vi "Initiate and Generate Time (Multi).vi"(0 "niUsrpRio Sessions":T3[](array[typedef]) {"Daughterboard Clock Rate" format="%#.3pHz"; "FPGA Data Clock Rate" format="%#.3pHz"; "Data Clock Rate" format="%#.3pHz"; "Characterization Data"."Frequencies [Hz]" format="%#_6p"; "EEPROM Characterization Header"."Pointer to Device Data Header" format="%x"; "EEPROM Characterization Header"."Checksum" format="%x"; "Device Data Header"."Pointer to Characterization Data" format="%x"; "Device Data Header"."Checksum" format="%x"; "EEPROM Header"."Pointer to User Header" format="%x"; "EEPROM Header"."Pointer to Factory Header" format="%x"; "EEPROM Header"."Product Code" format="%x"; "EEPROM Header"."Checksum" format="%x"}, 1 "tx channels":T1[](array[typedef]) {"tx.coerced configurations"."coerced sample rates" format="%#.3pS/s"; "tx.coerced configurations"."coerced levels" format="%#.3gdBm"; "tx.coerced configurations"."coerced lo frequencies" format="%#.3pHz"; "tx.coerced configurations"."coerced frequencies" format="%#.3pHz"; "tx config"."channel configuration"."channel configuration"."frequency" format="%#.3pHz"; "tx config"."channel configuration"."channel configuration"."lo frequency" format="%#.3pHz"; "tx config"."channel configuration"."channel configuration"."level" format="%#_gdBm"; "tx config"."tone frequency" format="%#.3pHz"; "tx config"."sample rate" format="%#.3pS/s"}, 5 "first iteration":bool, 7 "start trigger time":timestamp, 11 "error in":errorcluster) -> (4 "niUsrpRio Sessions (out)":T3[](array[typedef]) {"Daughterboard Clock Rate" format="%#.3pHz"; "FPGA Data Clock Rate" format="%#.3pHz"; "Data Clock Rate" format="%#.3pHz"; "Characterization Data"."Frequencies [Hz]" format="%#_6p"; "EEPROM Characterization Header"."Pointer to Device Data Header" format="%x"; "EEPROM Characterization Header"."Checksum" format="%x"; "Device Data Header"."Pointer to Characterization Data" format="%x"; "Device Data Header"."Checksum" format="%x"; "EEPROM Header"."Pointer to User Header" format="%x"; "EEPROM Header"."Pointer to Factory Header" format="%x"; "EEPROM Header"."Product Code" format="%x"; "EEPROM Header"."Checksum" format="%x"}, 15 "error out":errorcluster)   [LabVIEW 2020]
doc: "Writes baseband waveform to the device then initiates generation.\n\nVIs that must execute before this VI:\nOpen and Configure.vi\n\n<B>Input Parameters</B>\n\n<B>niUsrpRio Session</B> is the object created by the Open VI and used as the session handle for the USRP RIO design library.\n\n<B>first iteration</B> is used to determine if the device needs to be triggered. If this VI is in a loop, wire the iteration count to Equals Zero and then to this terminal. If this VI is not in a loop, wire a TRUE constant to this this terminal.\n\n<B>start trigger time</B> specifies the absolute time to initiate the start trigger. Only applies when the start trigger is set to Future Event.\n\n<B>error in</B> describes error conditions that occur before this node runs. This input provides standard 'error in' functionality.\n\n<B>Output Parameters</B>\n\n<B>niUsrpRio Session (out)</B> is the niUsrpRio session used in all subsequent USRP RIO design library host VIs.\n\n<B>error out</B> contains error information. This output provides standard 'error out' functionality."
uses:
  <instrlib>/niUsrpRio/Config/v1/Host/Public/niUsrpRio Session.ctl
  <instrlib>/_niInstr/Register Bus/v0/Host/Public/Register Bus Session.ctl
  <instrlib>/_niInstr/Register Bus/v0/Host/Private/Session Data.ctl
  <instrlib>/niUsrpRio/Config/v1/Host/Private/DB Queue Reference.ctl
  <instrlib>/niUsrpRio/Config/v1/Host/Private/Daughterboard Data.ctl
  <instrlib>/niUsrpRio/Config/v1/Host/Private/ATR state data.ctl
  <instrlib>/niUsrpRio/Config/v1/Host/Private/Antenna Configuration.ctl
  <instrlib>/niUsrpRio/Config/v1/Host/Private/CPLD Power Mode.ctl
  <instrlib>/niUsrpRio/Config/v1/Host/Public/EEPROM Header.ctl
  <instrlib>/niUsrpRio/Config/v1/Host/Public/EEPROM Device Data Header.ctl
  <instrlib>/niUsrpRio/Config/v1/Host/Public/EEPROM Characterization Header.ctl
  <instrlib>/niUsrpRio/Config/v1/Host/Public/Characterization Data.ctl
  <instrlib>/niUsrpRio/Config/v1/Host/Public/IQ Imbalance.ctl
  Tx Channels.ctl
  Start Trigger.ctl
  Write Tx Data (I16 multi).vi
  <instrlib>/_niInstr/Register Bus/v0/Host/niInstr Register Bus v0 Host.lvlib
  <instrlib>/niUsrpRio/Config/v1/Host/niUsrpRio Config v1 Host.lvlib
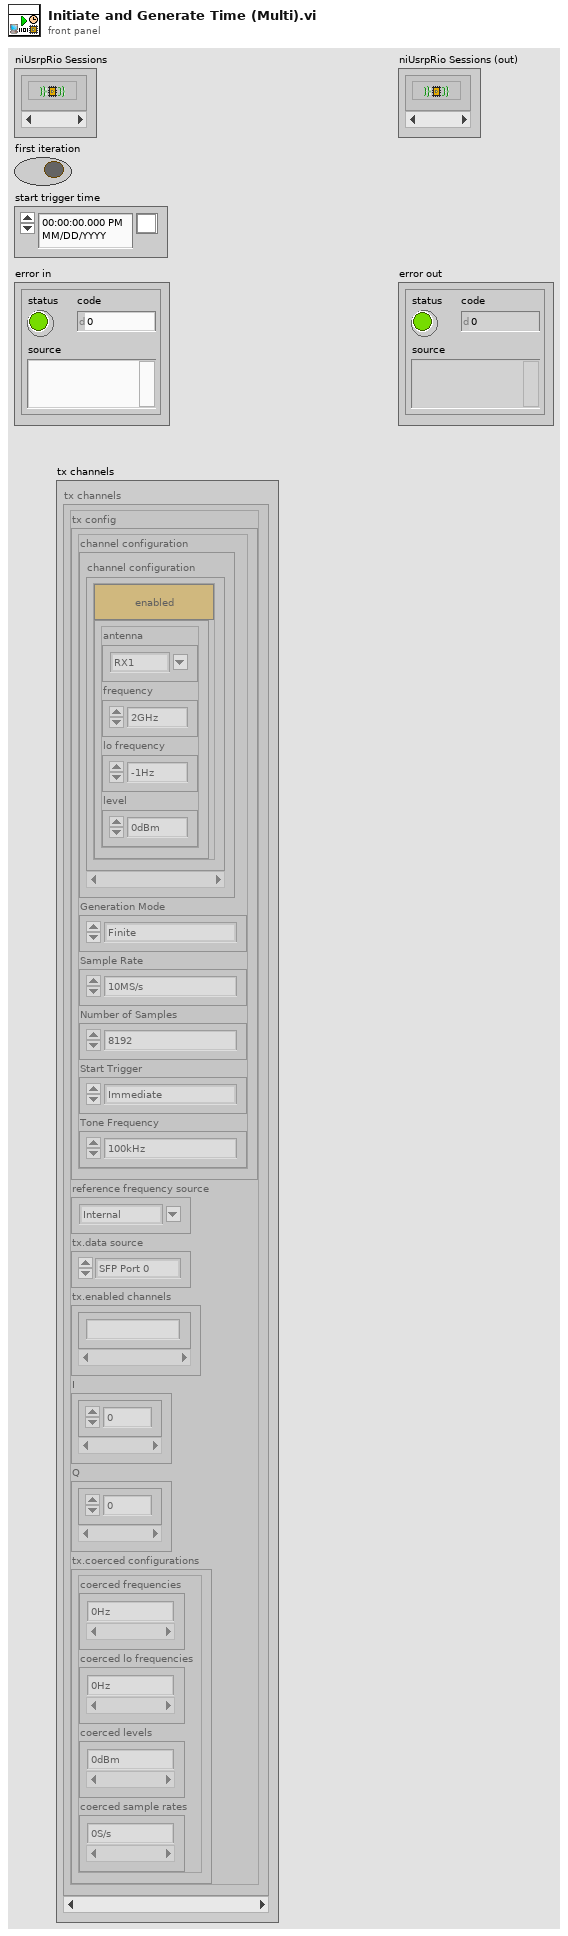
[diagram p1: front panel]
types:
  T1 = typedef "Tx Channels.ctl" = cluster{"tx config":cluster{"channel configuration":cluster{"channel enable":bool, "channel configuration":cluster{"antenna":string, "frequency":dbl, "lo frequency":dbl, "level":dbl}}[], "transfer mode":enum16{"Finite", "Continuous"}, "sample rate":dbl, "number of samples":u32, "start trigger":T2, "tone frequency":dbl}, "reference frequency source":string, "tx.data source":enum16{"SFP Port 0", "SFP Port 1", "Host"}, "tx.enabled channels":string[], "I":i16[], "Q":i16[], "tx.coerced configurations":cluster{"coerced frequencies":dbl[], "coerced lo frequencies":dbl[], "coerced levels":dbl[], "coerced sample rates":dbl[]}}
  T2 = typedef "Start Trigger.ctl" = enum8{"Software", "Digital Edge", "Rx Start Trigger", "Tx Start Trigger", "Immediate", "Future Time Event"}
  T3 = typedef "niUsrpRio Config v1 Host.lvlib/niUsrpRio Session.ctl" = cluster{"FPGA Interface":refnum<k20>, "RIO Interface Number":u32, "Data Clock Rate":u32, "FPGA Data Clock Rate":u32, "Global Settings Register Bus":T4, "Radio 0 Settings Register Bus":T4, "Radio 1 Settings Register Bus":T4, "Radio Settings Bus Semaphore":T5, "DB Queues":T6[], "Characterization Data Valid?":bool, "EEPROM Header":T7, "Device Data Header":T8, "EEPROM Characterization Header":T9, "Characterization Data":T10[], "FPGA Current Version":u32, "FPGA Oldest Compatible Version":u32, "Fixed Logic Current Version":u32, "Fixed Logic Oldest Compatible Version":u32, "FPGA Radio Settings Bus Current Version":u32, "FPGA Radio Settings Bus Oldest Compatible Version":u32, "FPGA Board Config Current Version":u32, "FPGA Board Config Oldest Compatible Version":u32, "Daughterboard Clock Rate":u32, "daughterboard configuration session handles":u64[]}
  T4 = typedef "niInstr Register Bus v0 Host.lvlib/Register Bus Session.ctl" = refnum<queue>
  T5 = typedef "Semaphore RefNum" = refnum<k1>
  T6 = typedef "niUsrpRio Config v1 Host.lvlib/DB Queue Reference.ctl" = refnum<queue>
  T7 = typedef "niUsrpRio Config v1 Host.lvlib/EEPROM Header.ctl" = cluster{"Checksum":u32, "Product Code":u16, "Hardware Current Version":u16, "Hardware Oldest Compatible Version":u16, "EEPROM Map Current Version":u16, "EEPROM Map Oldest Compatible Version":u16, "User Password":string, "Pointer to Factory Header":u32, "Pointer to User Header":u32, "Recommended Interval":u16, "Number of Reserved Bytes":i32, "Number of Daughterboards":u8, "Daughterboard IDs":u16[], "Daughterboard Serial Numbers":string[]}
  T8 = typedef "niUsrpRio Config v1 Host.lvlib/EEPROM Device Data Header.ctl" = cluster{"Checksum":u32, "Number of Channels":u8, "Number of Gain Settings":u16[], "Pointer to Characterization Data":u32[], "Number of Reserved Bytes":i32, "Number of Frequencies":u16[]}
  T9 = typedef "niUsrpRio Config v1 Host.lvlib/EEPROM Characterization Header.ctl" = cluster{"Checksum":u32, "Date":timestamp, "Temperature":sgl, "Misc. Info":string, "Pointer to Device Data Header":u32, "Number of Reserved Bytes":i32}
  T10 = typedef "niUsrpRio Config v1 Host.lvlib/Characterization Data.ctl" = cluster{"Gains[dB]":dbl[], "Frequencies [Hz]":dbl[], "IQ Imbalance Table":T11[], "Measured Gains[dB]":dbl[][]}
  T11 = typedef "niUsrpRio Config v1 Host.lvlib/IQ Imbalance.ctl" = cluster{"Gain Imbalance [linear]":dbl, "Phase Imbalance [radians]":dbl, "Offset":cdb}
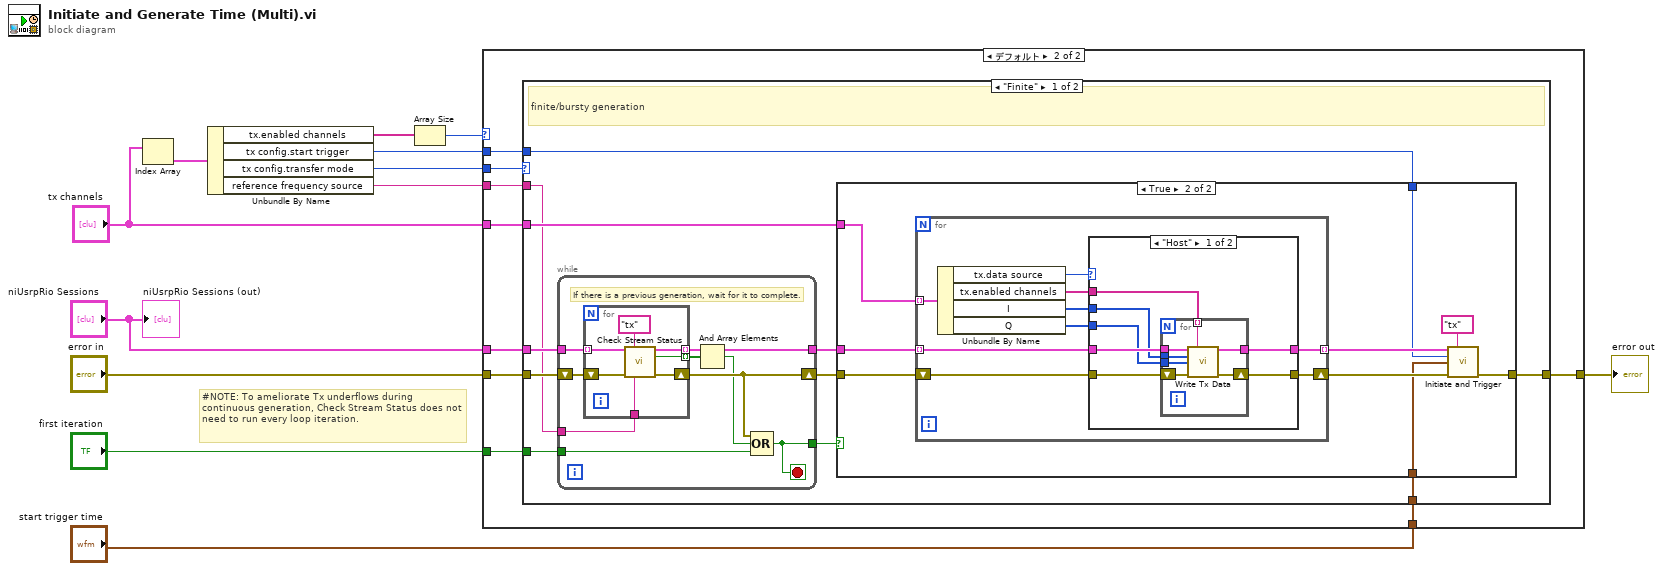
[diagram p0: block diagram]
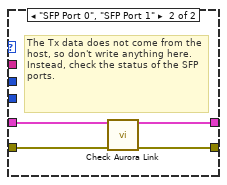
[diagram p4: hidden frame]
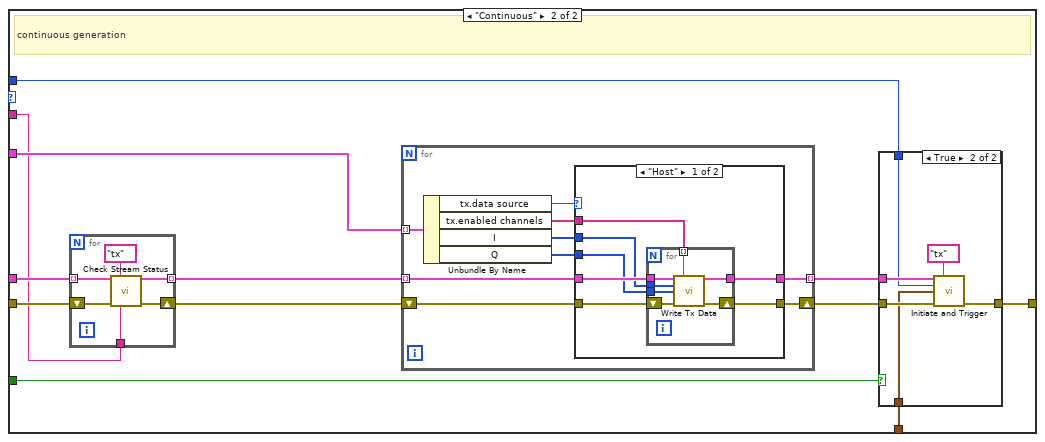
[diagram p5: hidden frame]
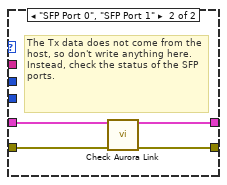
[diagram p7: hidden frame]
diagram:
  # "#NOTE: To ameliorate Tx underflows during continuous generation, Check Stream Status does not need to run every loop iteration."
  n1 = Index Array(array="tx channels") -> (element=w9:T1)  [unwired: 1 in]
  n2 = Unbundle By Name(w9) -> ("tx.enabled channels"=w5:string[], "tx config.start trigger"=w6:T2, "tx config.transfer mode"=w10:enum16{"Finite", "Continuous"}, "reference frequency source"=w7:string)
  n3 = Array Size(array=w5) -> (size(s)=w4:i32)
  n4 = case shown="デフォルト" w4 {
    tunnel: "niUsrpRio Sessions" -> [_ w22]
    tunnel: "error in" -> [w13 w21]
    tunnel: [w13 w20] -> w11
    tunnel: "first iteration" -> [_ w16]
    tunnel: w10 -> [_ w19]
    tunnel: "tx channels" -> [_ w18]
    tunnel: w7 -> [_ w14]
    tunnel: w6 -> [_ w17]
    tunnel: "start trigger time" -> [_ w15]
    frame 0 {
      # "do nothing if there are zero enabled channels"
    }
    frame Default {
      n5 = case shown="\"Finite\"" w19 {
        tunnel: w22 -> [w24 w91]
        tunnel: w21 -> [w25 w90]
        tunnel: [w33 w98] -> w20
        tunnel: w18 -> [w32 w97]
        tunnel: w17 -> [w31 w96]
        tunnel: w16 -> [w30 w93]
        tunnel: w14 -> [w23 w87]
        tunnel: w15 -> [w28 w92]
        frame "Finite" {
          # "finite/bursty generation"
          n6 = while {
            tunnel: w23 -> [w36]
            shift-right: [w42] -> w27
            shift-left: w25 -> [w39]
            tunnel: w30 -> [w41]
            tunnel: [w34] -> w29
            tunnel: w24 -> [w38]
            tunnel: [w35] -> w26
            stop <- w34 stop-if-true
            # "If there is a previous generation, wait for it to complete."
            n7 = for {
              tunnel: [w49] -> w40 mode=indexing
              shift-right: [w48] -> w42
              shift-left: w39 -> [w47]
              tunnel: w38 -> [w46] mode=indexing
              tunnel: [w45] -> w35 mode=indexing
              tunnel: w36 -> [w43]
              n8 = call "Check Stream Status.vi"("niUsrpRio Session"=w46, "scope"="tx", "error in"=w47, "reference frequency source"=w43) -> ("niUsrpRio Session (out)"=w45:T3, "done"=w49:bool, "error out"=w48:errorcluster)  [unwired: 9 in]
            }
            n9 = And Array Elements(Boolean array=w40) -> (logical AND=w37:bool)
            n10 = Compound Arithmetic op=OR(w42, w37, w41) -> (w34:bool)
          }
          n11 = case shown="TRUE" w29 {
            tunnel: w26 -> [_ w59]
            tunnel: w27 -> [w50 w58]
            tunnel: [w50 w55] -> w33
            tunnel: w32 -> [_ w56]
            tunnel: w31 -> [_ w52]
            tunnel: w28 -> [_ w51]
            frame False {
              # "Do nothing until the previous finite generation finishes before reinitiating."
            }
            frame True {
              n12 = for {
                tunnel: [w65] -> w54 mode=indexing
                tunnel: w59 -> [w67] mode=indexing
                shift-right: [w66] -> w57
                shift-left: w58 -> [w68]
                tunnel: w56 -> [w63] mode=indexing
                n13 = Unbundle By Name(w63) -> ("tx.data source"=w60:enum16{"SFP Port 0", "SFP Port 1", "Host"}, "tx.enabled channels"=w64:string[], "I"=w62:i16[], "Q"=w61:i16[])
                n14 = case shown="\"Host\"" w60 {
                  tunnel: w68 -> [w75 w84]
                  tunnel: w67 -> [w74 w86]
                  tunnel: [w73 w83] -> w66
                  tunnel: [w72 w85] -> w65
                  tunnel: w64 -> [w71 _]
                  tunnel: w62 -> [w70 _]
                  tunnel: w61 -> [w69 _]
                  frame "Host" {
                    n15 = for {
                      shift-right: [w81] -> w73
                      shift-left: w75 -> [w82]
                      tunnel: w74 -> [w80]
                      tunnel: [w79] -> w72
                      tunnel: w71 -> [w78] mode=indexing
                      tunnel: w70 -> [w77]
                      tunnel: w69 -> [w76]
                      n16 = call-poly "Write Tx Data.vi"("niUsrpRio Session"=w80, "scope"=w78, "I"=w77, "Q"=w76, "error in"=w82) -> ("niUsrpRio Session (out)"=w79:T3, "error out"=w81:errorcluster)  [unwired: 9 in]
                    }
                  }
                  frame "SFP Port 0", "SFP Port 1" {
                    # "The Tx data does not come from the host, so don't write anything here. Instead, check the status of the SFP ports."
                    n17 = call "Check Aurora Link.vi"("niUsrpRio Session"=w86, "error in"=w84) -> ("niUsrpRio Session (out)"=w85:T3, "error out"=w83:errorcluster)  [unwired: 12 in]
                  }
                }
              }
              n18 = call "Initiate and Trigger.vi"("niUsrpRio Sessions"=w54, "scope"="tx", "start trigger"=w52, "start trigger time"=w51, "error in"=w57) -> ("error out"=w55:errorcluster)  [unwired: 9 in, 1 out]
            }
          }
        }
        frame "Continuous" {
          # "continuous generation"
          n19 = for {
            shift-right: [w104] -> w88
            shift-left: w90 -> [w103]
            tunnel: w91 -> [w102] mode=indexing
            tunnel: [w101] -> w89 mode=indexing
            tunnel: w87 -> [w99]
            n20 = call "Check Stream Status.vi"("niUsrpRio Session"=w102, "scope"="tx", "error in"=w103, "reference frequency source"=w99) -> ("niUsrpRio Session (out)"=w101:T3, "error out"=w104:errorcluster)  [unwired: 9 in, 1 out]
          }
          n21 = for {
            tunnel: [w117] -> w94 mode=indexing
            tunnel: w89 -> [w119] mode=indexing
            shift-right: [w118] -> w95
            shift-left: w88 -> [w120]
            tunnel: w97 -> [w115] mode=indexing
            n22 = Unbundle By Name(w115) -> ("tx.data source"=w112:enum16{"SFP Port 0", "SFP Port 1", "Host"}, "tx.enabled channels"=w116:string[], "I"=w114:i16[], "Q"=w113:i16[])
            n23 = case shown="\"Host\"" w112 {
              tunnel: w120 -> [w127 w136]
              tunnel: w119 -> [w126 w138]
              tunnel: [w125 w135] -> w118
              tunnel: [w124 w137] -> w117
              tunnel: w116 -> [w123 _]
              tunnel: w114 -> [w122 _]
              tunnel: w113 -> [w121 _]
              frame "Host" {
                n24 = for {
                  shift-right: [w133] -> w125
                  shift-left: w127 -> [w134]
                  tunnel: w126 -> [w132]
                  tunnel: [w131] -> w124
                  tunnel: w123 -> [w130] mode=indexing
                  tunnel: w122 -> [w129]
                  tunnel: w121 -> [w128]
                  n25 = call-poly "Write Tx Data.vi"("niUsrpRio Session"=w132, "scope"=w130, "I"=w129, "Q"=w128, "error in"=w134) -> ("niUsrpRio Session (out)"=w131:T3, "error out"=w133:errorcluster)  [unwired: 9 in]
                }
              }
              frame "SFP Port 0", "SFP Port 1" {
                # "The Tx data does not come from the host, so don't write anything here. Instead, check the status of the SFP ports."
                n26 = call "Check Aurora Link.vi"("niUsrpRio Session"=w138, "error in"=w136) -> ("niUsrpRio Session (out)"=w137:T3, "error out"=w135:errorcluster)  [unwired: 12 in]
              }
            }
          }
          n27 = case shown="TRUE" w93 {
            tunnel: [w105 w110] -> w98
            tunnel: w96 -> [_ w109]
            tunnel: w95 -> [w105 w108]
            tunnel: w94 -> [_ w111]
            tunnel: w92 -> [_ w106]
            frame False {
              # "Only initiate on first iteration."
            }
            frame True {
              n28 = call "Initiate and Trigger.vi"("niUsrpRio Sessions"=w111, "scope"="tx", "start trigger"=w109, "start trigger time"=w106, "error in"=w108) -> ("error out"=w110:errorcluster)  [unwired: 9 in, 1 out]
            }
          }
        }
      }
    }
  }
  "error out" <- w11
  "niUsrpRio Sessions (out)" <- "niUsrpRio Sessions"
